vi "motor power and rpm.vi"(8 "error in (no error)":errorcluster, 9 "Motor":i16, 11 "data":waveform(dbl)[](array[waveform])) -> (0 "error out":errorcluster, 1 "Power":dbl, 2 "Phase to Phase Voltage":waveform(dbl), 4 "RPM":dbl, 5 "Phase Current":waveform(dbl))   [LabVIEW 2011]
uses:
  <vilib>/measure/madcrms.llb/Basic Averaged DC-RMS for 1 Chan.vi
  <vilib>/measure/NI_MAPro.lvlib
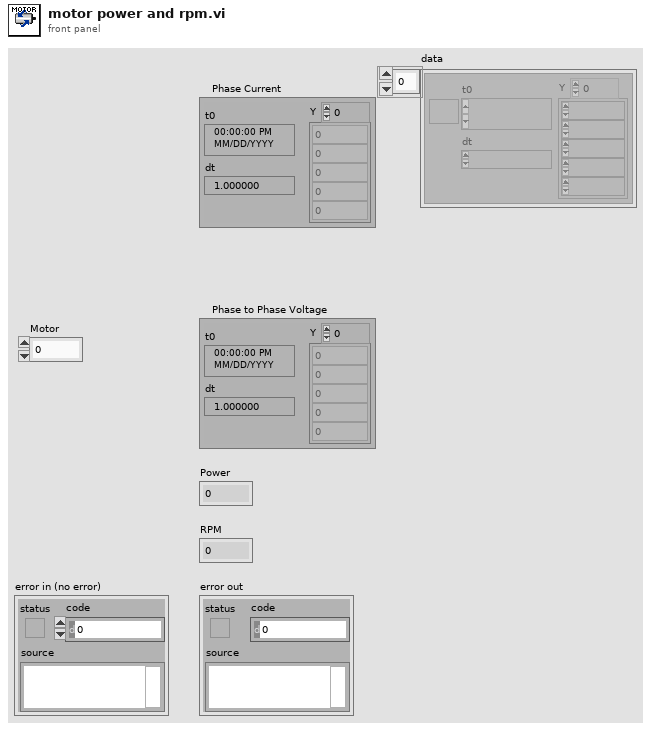
[diagram p1: front panel]
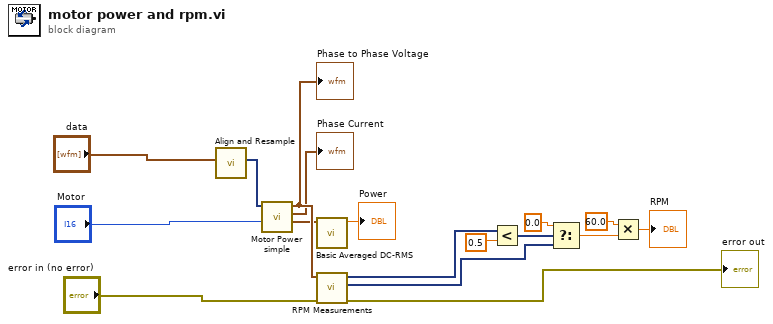
[diagram p0: block diagram]
diagram:
  n1 = call "Align and Resample"("Signals"="data") -> ("Resampled Signals"=w12:dynamicdata)  [unwired: 8 in, 2 out]
  n2 = call "Motor Power simple.vi"("Motor"="Motor", "data"=w12) -> ("Power"=w14:waveform(dbl), "Phase Current"=→"Phase Current":waveform(dbl), "Phase to Phase Voltage"=w17:waveform(dbl))  [unwired: 7 in]
  "Phase to Phase Voltage" <- w17
  n3 = call-poly <vilib>:"Basic Averaged DC-RMS.vi"("signal in"=w14) -> ("DC value"=→"Power":dbl)  [unwired: 7 in, 3 out]
  n4 = call "RPM Measurements"("error in (no error)"="error in (no error)", "Signals"=w17) -> ("error out"=→"error out":errorcluster, "Frequency"=w7:dynamicdata, "Amplitude"=w10:dynamicdata)  [unwired: 7 in]
  n5 = Less?(x=w10, y=0.5) -> (x < y?=w8:dynamicdata)
  n6 = Select(t=0.0, s=w8, f=w7) -> (s? t:f=w5:dbl)
  n7 = Multiply(x=60.0, y=w5) -> (x*y=→"RPM":dbl)
